vi "WrittingSpectrumAndImageAttributes.vi"() -> ()   [LabVIEW 2009]
uses:
  tango_lv8/tango_vi.llb/WriteBooleanSpectrumAttribute.vi
  tango_lv8/tango_vi.llb/WriteUShortSpectrumAttribute.vi
  tango_lv8/tango_vi.llb/WriteShortSpectrumAttribute.vi
  tango_lv8/tango_vi.llb/WriteUCharSpectrumAttribute.vi
  tango_lv8/tango_vi.llb/ReadShortImageAttribute.vi
  tango_lv8/tango_vi.llb/WriteShortImageAttribute.vi
  tango_lv8/tango_vi.llb/WriteFloatSpectrumAttribute.vi
  tango_lv8/tango_vi.llb/WriteDoubleSpectrumAttribute.vi
  tango_lv8/tango_vi.llb/WriteLongSpectrumAttribute.vi
  tango_lv8/tango_vi.llb/ReadLongImageAttribute.vi
  tango_lv8/tango_vi.llb/WriteLongImageAttribute.vi
  tango_lv8/tango_vi.llb/ReadUShortImageAttribute.vi
  tango_lv8/tango_vi.llb/WriteUShortImageAttribute.vi
  tango_lv8/tango_vi.llb/ReadUCharImageAttribute.vi
  tango_lv8/tango_vi.llb/WriteUCharImageAttribute.vi
  tango_lv8/tango_vi.llb/ReadBooleanImageAttribute.vi
  tango_lv8/tango_vi.llb/WriteBooleanImageAttribute.vi
  tango_lv8/tango_vi.llb/ReadFloatImageAttribute.vi
  tango_lv8/tango_vi.llb/WriteFloatImageAttribute.vi
  tango_lv8/tango_vi.llb/ReadDoubleImageAttribute.vi
  tango_lv8/tango_vi.llb/WriteDoubleImageAttribute.vi
  tango_lv8/tango_vi.llb/ReadBooleanSpectrumAttribute.vi
  tango_lv8/tango_vi.llb/ReadUCharSpectrumAttribute.vi
  tango_lv8/tango_vi.llb/ReadUShortSpectrumAttribute.vi
  tango_lv8/tango_vi.llb/ReadShortSpectrumAttribute.vi
  tango_lv8/tango_vi.llb/ReadFloatSpectrumAttribute.vi
  tango_lv8/tango_vi.llb/ReadDoubleSpectrumAttribute.vi
  tango_lv8/tango_vi.llb/ReadLongSpectrumAttribute.vi
  tango_lv8/tango_vi.llb/ReadULongImageAttribute.vi
  tango_lv8/tango_vi.llb/WriteULongImageAttribute.vi
  tango_lv8/tango_vi.llb/WriteULongSpectrumAttribute.vi
  tango_lv8/tango_vi.llb/ReadULongSpectrumAttribute.vi
panel:
  out "ULong Spectrum R":u32[](graph)
  out "Success-R":bool
  out "Success-Cmp 4":bool
  out "Success-W":bool
  out "ULong  Spectrum W":u32[](graph)
  in  "TangoTest dev. name 3":string="tango/tangotest/1"
  out "Success-R":bool
  out "Success-Cmp 3":bool
  out "ULong Image R":u32[][](graph)
  out "Success-W":bool
  out "ULong Image W":u32[][](graph)
  out "Success-R":bool
  out "Success-Cmp":bool
  out "Double  Image R":dbl[][](graph)
  out "Success-W":bool
  out "Double Image W":dbl[][](graph)
  out "Success-R":bool
  out "Success-Cmp":bool
  out "Float Image R":sgl[][](graph)
  out "Success-W":bool
  out "Float Image W":sgl[][](graph)
  out "Success-R":bool
  out "Success-Cmp":bool
  out "Boolean  Image R":i16[][](graph)
  out "Success-W":bool
  out "Boolean Image W":i16[][](graph)
  out "Success-R":bool
  out "Success-Cmp":bool
  out "UChar Image R":u8[][](graph)
  out "Success-W":bool
  out "UChar Image W":u8[][](graph)
  out "Success-R":bool
  out "Success-Cmp":bool
  out "UShort Image R":u16[][](graph)
  out "Success-W":bool
  out "UShort Image W":u16[][](graph)
  out "Long Spectrum R":i32[](graph)
  out "Success-R":bool
  out "Success-Cmp":bool
  out "Success-W":bool
  out "Long  Spectrum W":i32[](graph)
  out "Success-R":bool
  out "Success-Cmp":bool
  out "Long Image R":i32[][](graph)
  out "Success-W":bool
  out "Long Image W":i32[][](graph)
  out "Double Spectrum R":dbl[](graph)
  out "Success-R":bool
  out "Success-Cmp":bool
  out "Success-W":bool
  out "Double  Spectrum W":dbl[](graph)
  out "Float Spectrum R":sgl[](graph)
  out "Success-R":bool
  out "Success-Cmp":bool
  out "Success-W":bool
  out "Float Spectrum W":sgl[](graph)
  out "Short Image R":i16[][](graph)
  out "Short Image W":i16[][](graph)
  out "Success-R":bool
  out "Success-Cmp 2":bool
  out "Success-W":bool
  out "error stack":string[](array[string])
  in  "TangoTest Device Name 5":string="tango/tangotest/1"
  in  "TangoTest Device Name 4":string="tango/tangotest/1"
  in  "TangoTest Device Name 3":string="tango/tangotest/1"
  in  "TangoTest Device Name 2":string="tango/tangotest/1"
  in  "TangoTest dev. name":string="tango/tangotest/1"
  out "UChar Spectrum R":u8[](graph)
  out "Success-R":bool
  out "Success-Cmp":bool
  out "Success-W":bool
  out "UChar Spectrum W":u8[](graph)
  out "Boolean Spectrum R":i16[](graph)
  out "Success-R":bool
  out "Success-Cmp":bool
  out "Success-W":bool
  out "Boolean Spectrum W":i16[](graph)
  out "UShort Spectrum R":u16[](graph)
  out "Success-R":bool
  out "Success-Cmp":bool
  out "Success-W":bool
  out "UShort Spectrum W":u16[](graph)
  out "Success-Cmp":bool
  out "Success-W":bool
  out "Short Spectrum R":i16[](graph)
  out "Success-R":bool
  out "Short Spectrum W":i16[](graph)
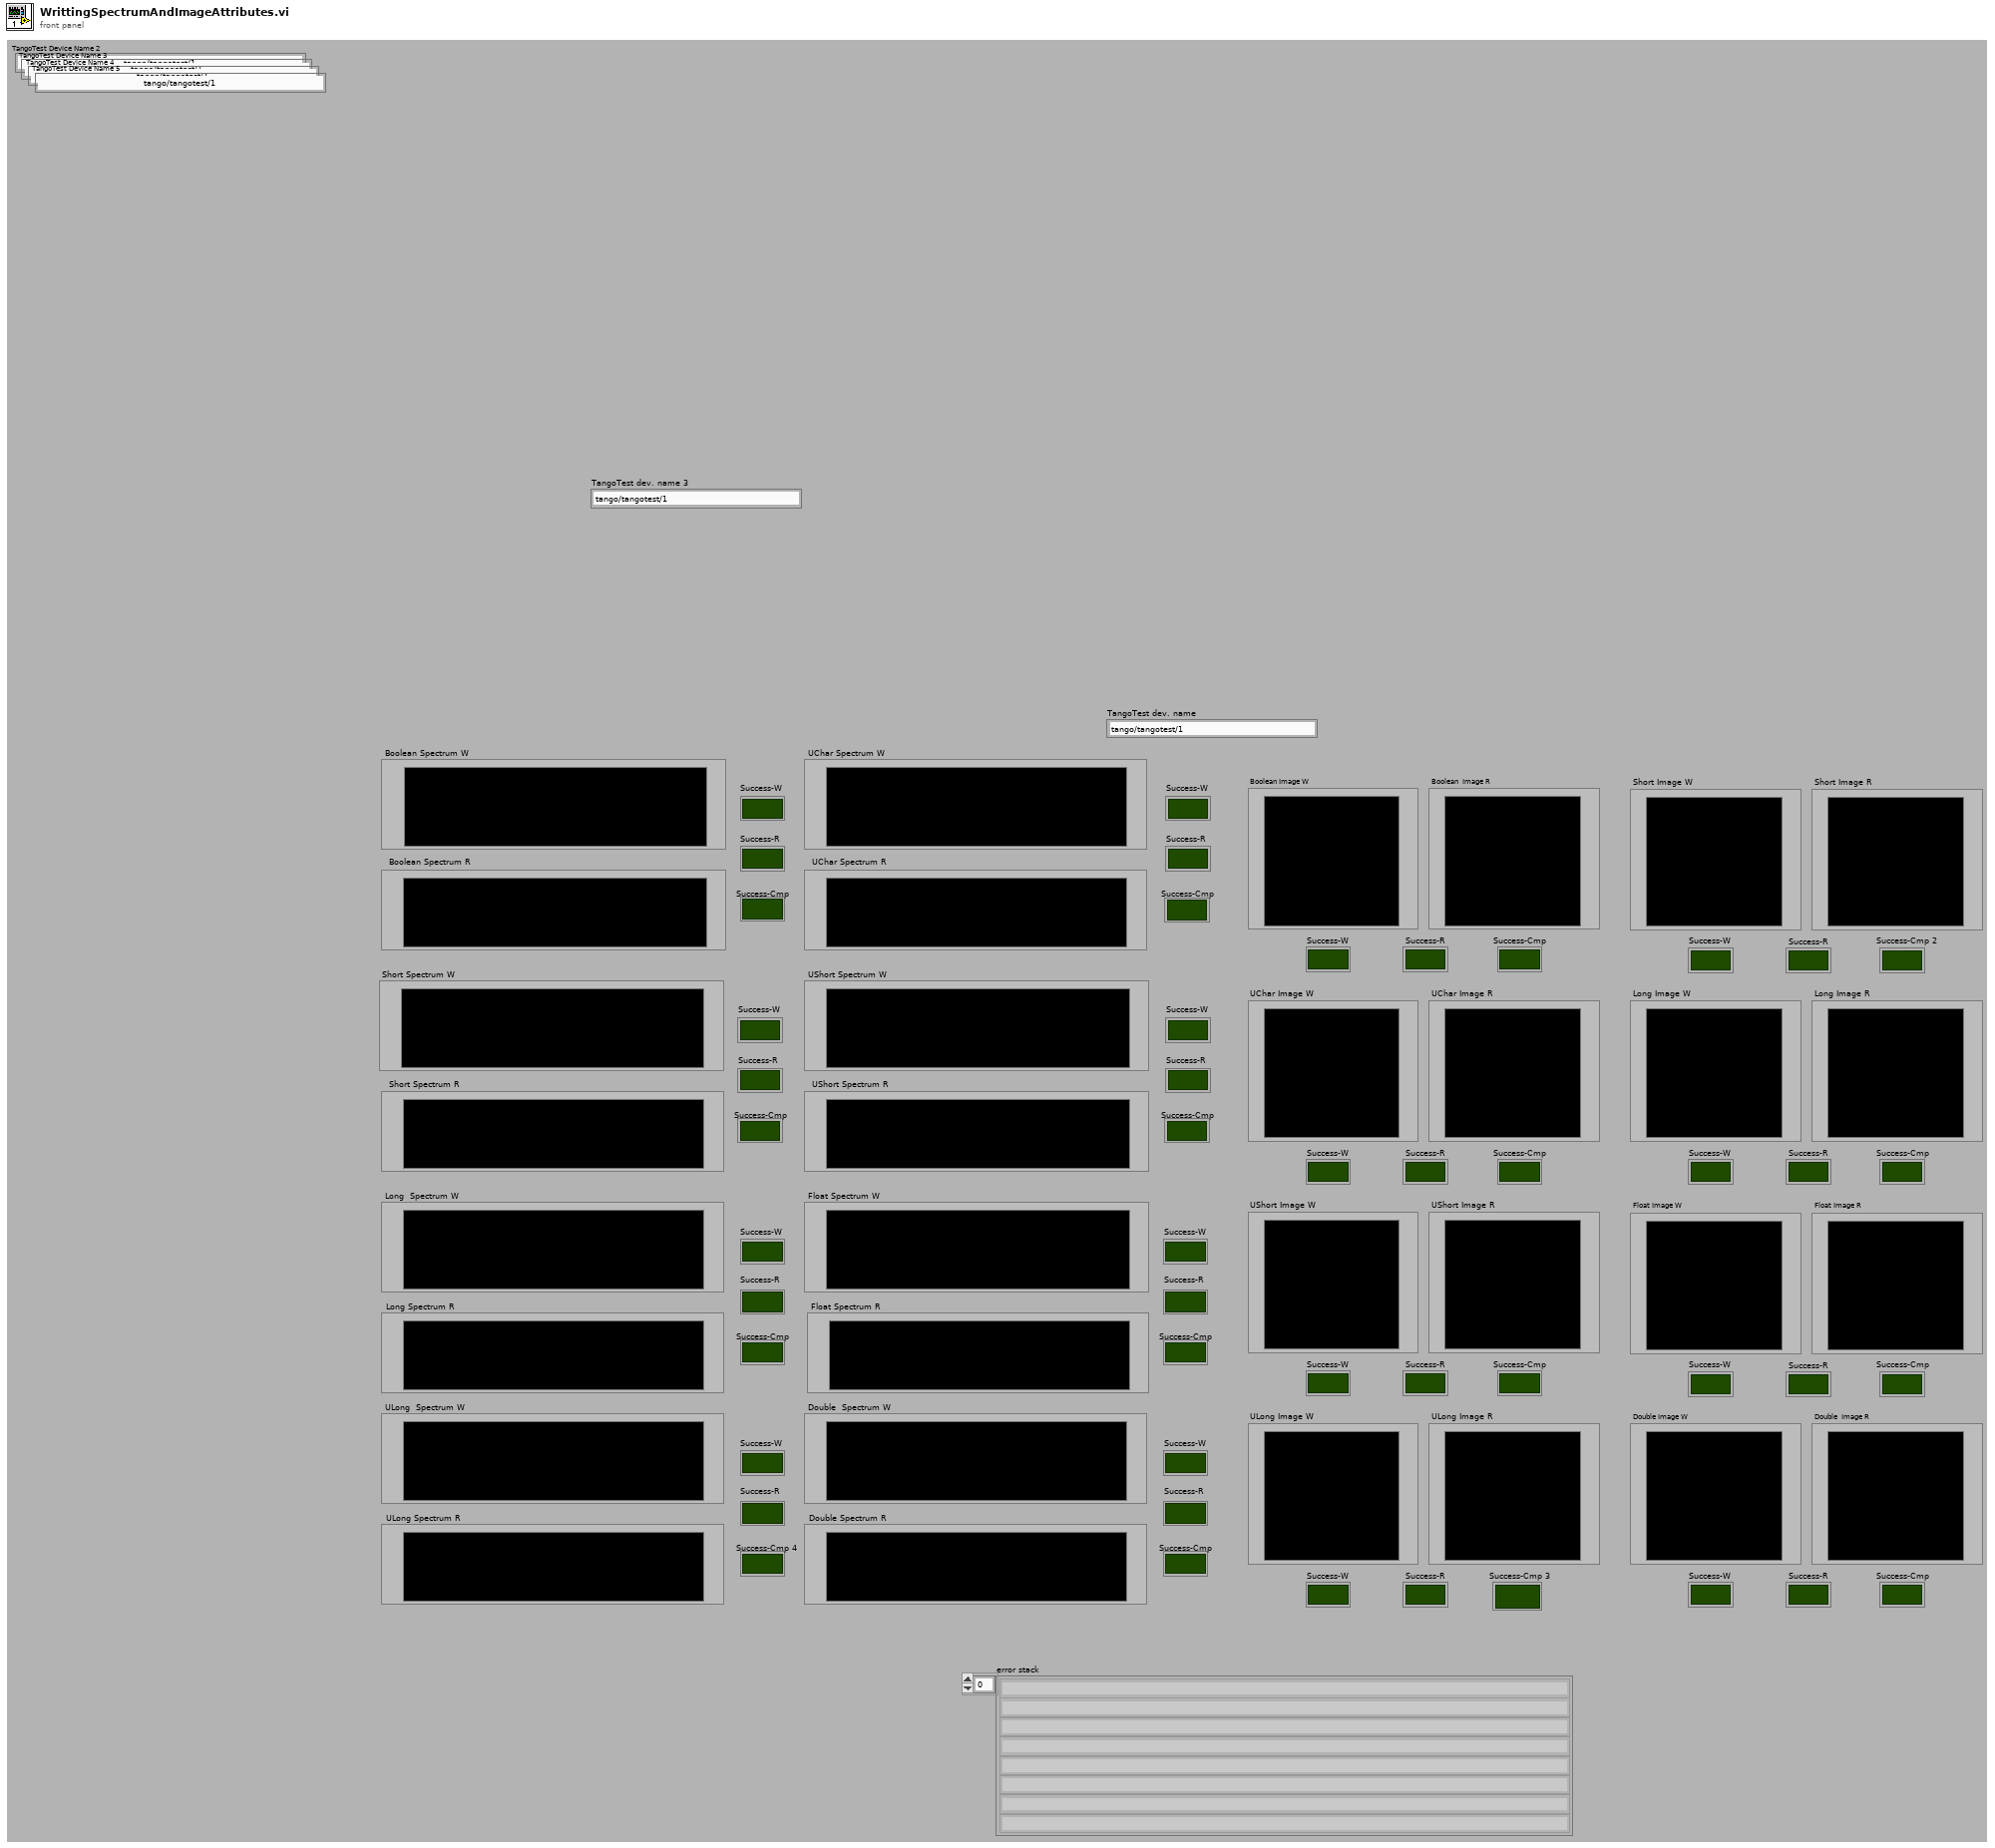
[diagram p1: front panel]
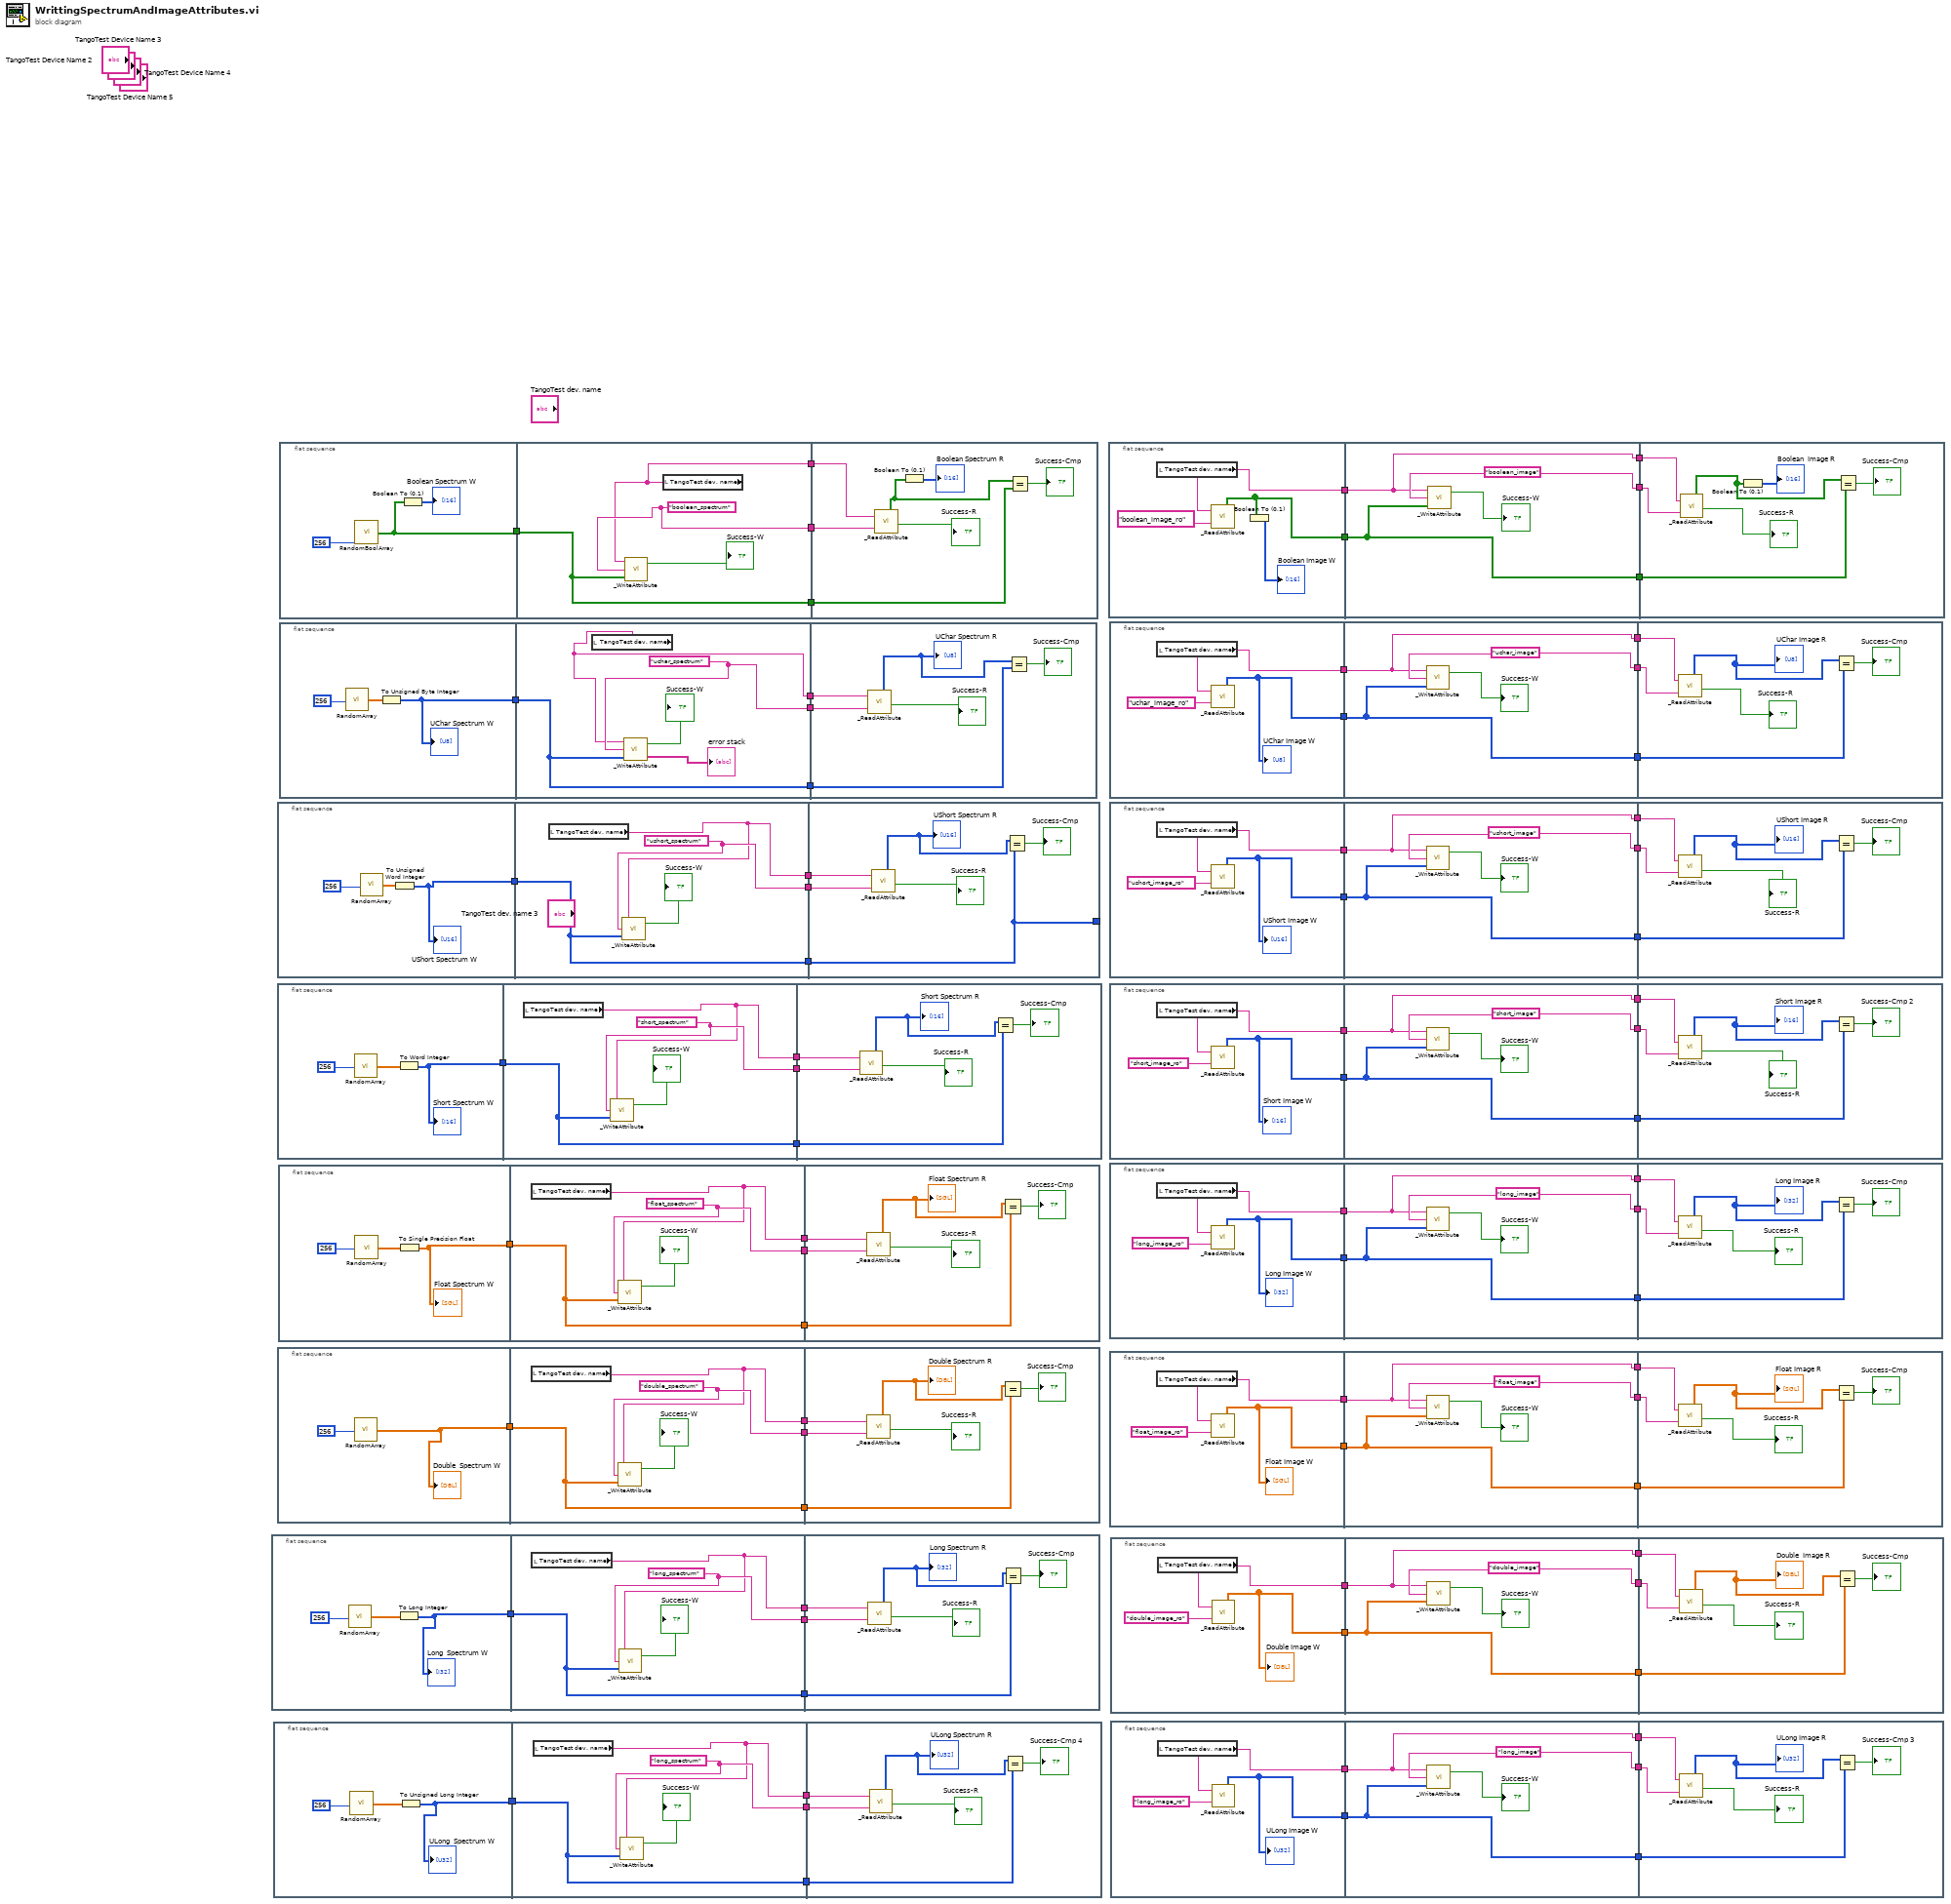
[diagram p0: block diagram]
diagram:
  n1 = flat-sequence {
    tunnel: [w73] -> w38
    tunnel: [w76] -> w37
    tunnel: [w78] -> w36
    tunnel: [w77] -> w35
    tunnel: w38 -> [w77]
    tunnel: w37 -> [w84]
    tunnel: w36 -> [w83]
    tunnel: w35 -> [w81]
    frame #0 {
      n2 = call "RandomArray.vi"("random array size"=256) -> ("random array"=w74:dbl[])  [unwired: 1 in]
      n3 = To Long Integer(number=w74) -> (32bit integer=w73:i32[])
      "Long  Spectrum W" <- w73
    }
    frame #1 {
      w78 = "long_spectrum" ("attribute name")
      n4 = local read "TangoTest dev. name"() -> (w76:string)
      n5 = call-poly "_WriteAttribute.vi"("value"=w77, "attribute name"=w78, "device name"=w76) -> ("success"=→"Success-W":bool)  [unwired: 1 out]
    }
    frame #2 {
      n6 = call-poly "_ReadAttribute.vi"("device name"=w84, "attribute name"=w83) -> ("value"=w82:i32[], "success"=→"Success-R":bool)  [unwired: 4 out]
      "Long Spectrum R" <- w82
      n7 = Equal?(x=w82, y=w81) -> (x = y?=→"Success-Cmp":bool)
    }
  }
  n8 = flat-sequence {
    tunnel: [w86] -> w4
    tunnel: [w89] -> w3
    tunnel: [w91] -> w2
    tunnel: [w90] -> w1
    tunnel: w4 -> [w90]
    tunnel: w3 -> [w97]
    tunnel: w2 -> [w96]
    tunnel: w1 -> [w94]
    frame #0 {
      n9 = call "RandomArray.vi"("random array size"=256) -> ("random array"=w87:dbl[])  [unwired: 1 in]
      n10 = To Unsigned Long Integer(number=w87) -> (unsigned 32bit integer=w86:u32[])
      "ULong  Spectrum W" <- w86
    }
    frame #1 {
      w91 = "long_spectrum" ("attribute name")
      n11 = local read "TangoTest dev. name"() -> (w89:string)
      n12 = call-poly "_WriteAttribute.vi"("value"=w90, "attribute name"=w91, "device name"=w89) -> ("success"=→"Success-W":bool)  [unwired: 1 out]
    }
    frame #2 {
      n13 = call-poly "_ReadAttribute.vi"("device name"=w97, "attribute name"=w96) -> ("value"=w95:u32[], "success"=→"Success-R":bool)  [unwired: 4 out]
      "ULong Spectrum R" <- w95
      n14 = Equal?(x=w95, y=w94) -> (x = y?=→"Success-Cmp 4":bool)
    }
  }
  n15 = flat-sequence {
    tunnel: [w99] -> w68
    tunnel: [w102] -> w67
    tunnel: [w104] -> w66
    tunnel: [w103] -> w65
    tunnel: w68 -> [w103]
    tunnel: w67 -> [w110]
    tunnel: w66 -> [w109]
    tunnel: w65 -> [w106]
    tunnel: [w106] -> _
    frame #0 {
      n16 = call "RandomArray.vi"("random array size"=256) -> ("random array"=w100:dbl[])  [unwired: 1 in]
      n17 = To Unsigned Word Integer(number=w100) -> (unsigned 16bit integer=w99:u16[])
      "UShort Spectrum W" <- w99
    }
    frame #1 {
      w104 = "ushort_spectrum" ("attribute name")
      n18 = local read "TangoTest dev. name"() -> (w102:string)
      n19 = call-poly "_WriteAttribute.vi"("value"=w103, "attribute name"=w104, "device name"=w102) -> ("success"=→"Success-W":bool)  [unwired: 1 out]
    }
    frame #2 {
      n20 = call-poly "_ReadAttribute.vi"("device name"=w110, "attribute name"=w109) -> ("value"=w108:u16[], "success"=→"Success-R":bool)  [unwired: 4 out]
      "UShort Spectrum R" <- w108
      n21 = Equal?(x=w108, y=w106) -> (x = y?=→"Success-Cmp":bool)
    }
  }
  n22 = flat-sequence {
    tunnel: [w112] -> w69
    tunnel: [w115] -> w72
    tunnel: [w117] -> w71
    tunnel: [w116] -> w70
    tunnel: w69 -> [w116]
    tunnel: w72 -> [w123]
    tunnel: w71 -> [w122]
    tunnel: w70 -> [w120]
    frame #0 {
      n23 = call "RandomArray.vi"("random array size"=256) -> ("random array"=w113:dbl[])  [unwired: 1 in]
      n24 = To Word Integer(number=w113) -> (16bit integer=w112:i16[])
      "Short Spectrum W" <- w112
    }
    frame #1 {
      w117 = "short_spectrum" ("attribute name")
      n25 = local read "TangoTest dev. name"() -> (w115:string)
      n26 = call-poly "_WriteAttribute.vi"("value"=w116, "attribute name"=w117, "device name"=w115) -> ("success"=→"Success-W":bool)  [unwired: 1 out]
    }
    frame #2 {
      n27 = call-poly "_ReadAttribute.vi"("device name"=w123, "attribute name"=w122) -> ("value"=w121:i16[], "success"=→"Success-R":bool)  [unwired: 4 out]
      "Short Spectrum R" <- w121
      n28 = Equal?(x=w121, y=w120) -> (x = y?=→"Success-Cmp":bool)
    }
  }
  n29 = flat-sequence {
    tunnel: [w125] -> w47
    tunnel: [w127] -> w46
    tunnel: [w129] -> w45
    tunnel: [w128] -> w44
    tunnel: w47 -> [w128]
    tunnel: w46 -> [w135]
    tunnel: w45 -> [w134]
    tunnel: w44 -> [w132]
    frame #0 {
      n30 = call "RandomArray.vi"("random array size"=256) -> ("random array"=w125:dbl[])  [unwired: 1 in]
      "Double  Spectrum W" <- w125
    }
    frame #1 {
      w129 = "double_spectrum" ("attribute name")
      n31 = local read "TangoTest dev. name"() -> (w127:string)
      n32 = call-poly "_WriteAttribute.vi"("value"=w128, "attribute name"=w129, "device name"=w127) -> ("success"=→"Success-W":bool)  [unwired: 1 out]
    }
    frame #2 {
      n33 = call-poly "_ReadAttribute.vi"("device name"=w135, "attribute name"=w134) -> ("value"=w133:dbl[], "success"=→"Success-R":bool)  [unwired: 4 out]
      "Double Spectrum R" <- w133
      n34 = Equal?(x=w133, y=w132) -> (x = y?=→"Success-Cmp":bool)
    }
  }
  n35 = flat-sequence {
    tunnel: [w137] -> w51
    tunnel: [w140] -> w50
    tunnel: [w142] -> w49
    tunnel: [w141] -> w48
    tunnel: w51 -> [w141]
    tunnel: w50 -> [w148]
    tunnel: w49 -> [w147]
    tunnel: w48 -> [w145]
    frame #0 {
      n36 = call "RandomArray.vi"("random array size"=256) -> ("random array"=w138:dbl[])  [unwired: 1 in]
      n37 = To Single Precision Float(number=w138) -> (single precision float=w137:sgl[])
      "Float Spectrum W" <- w137
    }
    frame #1 {
      w142 = "float_spectrum" ("attribute name")
      n38 = local read "TangoTest dev. name"() -> (w140:string)
      n39 = call-poly "_WriteAttribute.vi"("value"=w141, "attribute name"=w142, "device name"=w140) -> ("success"=→"Success-W":bool)  [unwired: 1 out]
    }
    frame #2 {
      n40 = call-poly "_ReadAttribute.vi"("device name"=w148, "attribute name"=w147) -> ("value"=w146:sgl[], "success"=→"Success-R":bool)  [unwired: 4 out]
      "Float Spectrum R" <- w146
      n41 = Equal?(x=w146, y=w145) -> (x = y?=→"Success-Cmp":bool)
    }
  }
  n42 = flat-sequence {
    tunnel: [w150] -> w58
    tunnel: [w154] -> w62
    tunnel: [w156] -> w61
    tunnel: w58 -> [w155]
    tunnel: [w155] -> w57
    tunnel: w62 -> [w162]
    tunnel: w61 -> [w161]
    tunnel: w57 -> [w158]
    frame #0 {
      n43 = call "RandomArray.vi"("random array size"=256) -> ("random array"=w151:dbl[])  [unwired: 1 in]
      n44 = To Unsigned Byte Integer(number=w151) -> (unsigned 8bit integer=w150:u8[])
      "UChar Spectrum W" <- w150
    }
    frame #1 {
      w156 = "uchar_spectrum" ("attribute name")
      n45 = local read "TangoTest dev. name"() -> (w154:string)
      n46 = call-poly "_WriteAttribute.vi"("value"=w155, "attribute name"=w156, "device name"=w154) -> ("error stack"=→"error stack":string[], "success"=→"Success-W":bool)
    }
    frame #2 {
      n47 = call-poly "_ReadAttribute.vi"("device name"=w162, "attribute name"=w161) -> ("value"=w160:u8[], "success"=→"Success-R":bool)  [unwired: 4 out]
      "UChar Spectrum R" <- w160
      n48 = Equal?(x=w160, y=w158) -> (x = y?=→"Success-Cmp":bool)
    }
  }
  n49 = flat-sequence {
    tunnel: [w165] -> w64
    tunnel: [w169] -> w63
    tunnel: w64 -> [w169]
    tunnel: [w168] -> w60
    tunnel: [w167] -> w59
    tunnel: w63 -> [w173]
    tunnel: w60 -> [w172]
    tunnel: w59 -> [w171]
    frame #0 {
      n50 = call "RandomBoolArray.vi"("random array size"=256) -> ("random array"=w165:bool[])  [unwired: 1 in]
      n51 = Boolean To (0,1)(Boolean=w165) -> (0, 1=→"Boolean Spectrum W":i16[])
    }
    frame #1 {
      w168 = "boolean_spectrum" ("attribute name")
      n52 = local read "TangoTest dev. name"() -> (w167:string)
      n53 = call-poly "_WriteAttribute.vi"("value"=w169, "attribute name"=w168, "device name"=w167) -> ("success"=→"Success-W":bool)  [unwired: 1 out]
    }
    frame #2 {
      n54 = call-poly "_ReadAttribute.vi"("device name"=w171, "attribute name"=w172) -> ("value"=w175:bool[], "success"=→"Success-R":bool)  [unwired: 4 out]
      n55 = Boolean To (0,1)(Boolean=w175) -> (0, 1=→"Boolean Spectrum R":i16[])
      n56 = Equal?(x=w175, y=w173) -> (x = y?=→"Success-Cmp":bool)
    }
  }
  n57 = flat-sequence {
    tunnel: [w180] -> w24
    tunnel: [w179] -> w23
    tunnel: [w185] -> w22
    tunnel: [w183] -> w21
    tunnel: w24 -> [w183]
    tunnel: w23 -> [w182]
    tunnel: [w182] -> w20
    tunnel: w22 -> [w191]
    tunnel: w21 -> [w188]
    tunnel: w20 -> [w187]
    frame #0 {
      n58 = local read "TangoTest dev. name"() -> (w179:string)
      n59 = call-poly "_ReadAttribute.vi"("device name"=w179, "attribute name"="boolean_image_ro") -> ("value"=w180:bool[][])  [unwired: 5 out]
      n60 = Boolean To (0,1)(Boolean=w180) -> (0, 1=→"Boolean Image W":i16[][])
    }
    frame #1 {
      w185 = "boolean_image" ("attribute name")
      n61 = call-poly "_WriteAttribute.vi"("value"=w183, "attribute name"=w185, "device name"=w182) -> ("success"=→"Success-W":bool)  [unwired: 1 out]
    }
    frame #2 {
      n62 = call-poly "_ReadAttribute.vi"("device name"=w187, "attribute name"=w191) -> ("value"=w189:bool[][], "success"=→"Success-R":bool)  [unwired: 4 out]
      n63 = Boolean To (0,1)(Boolean=w189) -> (0, 1=→"Boolean  Image R":i16[][])
      n64 = Equal?(x=w189, y=w188) -> (x = y?=→"Success-Cmp":bool)
    }
  }
  n65 = flat-sequence {
    tunnel: [w194] -> w29
    tunnel: [w193] -> w28
    tunnel: [w199] -> w27
    tunnel: [w197] -> w26
    tunnel: w29 -> [w197]
    tunnel: w28 -> [w196]
    tunnel: [w196] -> w25
    tunnel: w27 -> [w204]
    tunnel: w26 -> [w201]
    tunnel: w25 -> [w200]
    frame #0 {
      n66 = local read "TangoTest dev. name"() -> (w193:string)
      n67 = call-poly "_ReadAttribute.vi"("device name"=w193, "attribute name"="uchar_image_ro") -> ("value"=w194:u8[][])  [unwired: 5 out]
      "UChar Image W" <- w194
    }
    frame #1 {
      w199 = "uchar_image" ("attribute name")
      n68 = call-poly "_WriteAttribute.vi"("value"=w197, "attribute name"=w199, "device name"=w196) -> ("success"=→"Success-W":bool)  [unwired: 1 out]
    }
    frame #2 {
      n69 = call-poly "_ReadAttribute.vi"("device name"=w200, "attribute name"=w204) -> ("value"=w202:u8[][], "success"=→"Success-R":bool)  [unwired: 4 out]
      "UChar Image R" <- w202
      n70 = Equal?(x=w202, y=w201) -> (x = y?=→"Success-Cmp":bool)
    }
  }
  n71 = flat-sequence {
    tunnel: [w207] -> w34
    tunnel: [w206] -> w33
    tunnel: [w212] -> w32
    tunnel: [w210] -> w31
    tunnel: w34 -> [w210]
    tunnel: w33 -> [w209]
    tunnel: [w209] -> w30
    tunnel: w32 -> [w217]
    tunnel: w31 -> [w214]
    tunnel: w30 -> [w213]
    frame #0 {
      n72 = local read "TangoTest dev. name"() -> (w206:string)
      n73 = call-poly "_ReadAttribute.vi"("device name"=w206, "attribute name"="ushort_image_ro") -> ("value"=w207:u16[][])  [unwired: 5 out]
      "UShort Image W" <- w207
    }
    frame #1 {
      w212 = "ushort_image" ("attribute name")
      n74 = call-poly "_WriteAttribute.vi"("value"=w210, "attribute name"=w212, "device name"=w209) -> ("success"=→"Success-W":bool)  [unwired: 1 out]
    }
    frame #2 {
      n75 = call-poly "_ReadAttribute.vi"("device name"=w213, "attribute name"=w217) -> ("value"=w215:u16[][], "success"=→"Success-R":bool)  [unwired: 4 out]
      "UShort Image R" <- w215
      n76 = Equal?(x=w215, y=w214) -> (x = y?=→"Success-Cmp":bool)
    }
  }
  n77 = flat-sequence {
    tunnel: [w220] -> w54
    tunnel: [w219] -> w53
    tunnel: [w225] -> w56
    tunnel: [w223] -> w55
    tunnel: w54 -> [w223]
    tunnel: w53 -> [w222]
    tunnel: [w222] -> w52
    tunnel: w56 -> [w230]
    tunnel: w55 -> [w227]
    tunnel: w52 -> [w226]
    frame #0 {
      n78 = local read "TangoTest dev. name"() -> (w219:string)
      n79 = call-poly "_ReadAttribute.vi"("device name"=w219, "attribute name"="short_image_ro") -> ("value"=w220:i16[][])  [unwired: 5 out]
      "Short Image W" <- w220
    }
    frame #1 {
      w225 = "short_image" ("attribute name")
      n80 = call-poly "_WriteAttribute.vi"("value"=w223, "attribute name"=w225, "device name"=w222) -> ("success"=→"Success-W":bool)  [unwired: 1 out]
    }
    frame #2 {
      n81 = call-poly "_ReadAttribute.vi"("device name"=w226, "attribute name"=w230) -> ("value"=w228:i16[][], "success"=→"Success-R":bool)  [unwired: 4 out]
      "Short Image R" <- w228
      n82 = Equal?(x=w228, y=w227) -> (x = y?=→"Success-Cmp 2":bool)
    }
  }
  n83 = flat-sequence {
    tunnel: [w233] -> w43
    tunnel: [w232] -> w42
    tunnel: [w238] -> w41
    tunnel: [w236] -> w40
    tunnel: w43 -> [w236]
    tunnel: w42 -> [w235]
    tunnel: [w235] -> w39
    tunnel: w41 -> [w243]
    tunnel: w40 -> [w240]
    tunnel: w39 -> [w239]
    frame #0 {
      n84 = local read "TangoTest dev. name"() -> (w232:string)
      n85 = call-poly "_ReadAttribute.vi"("device name"=w232, "attribute name"="long_image_ro") -> ("value"=w233:i32[][])  [unwired: 5 out]
      "Long Image W" <- w233
    }
    frame #1 {
      w238 = "long_image" ("attribute name")
      n86 = call-poly "_WriteAttribute.vi"("value"=w236, "attribute name"=w238, "device name"=w235) -> ("success"=→"Success-W":bool)  [unwired: 1 out]
    }
    frame #2 {
      n87 = call-poly "_ReadAttribute.vi"("device name"=w239, "attribute name"=w243) -> ("value"=w241:i32[][], "success"=→"Success-R":bool)  [unwired: 4 out]
      "Long Image R" <- w241
      n88 = Equal?(x=w241, y=w240) -> (x = y?=→"Success-Cmp":bool)
    }
  }
  n89 = flat-sequence {
    tunnel: [w246] -> w19
    tunnel: [w245] -> w18
    tunnel: [w251] -> w17
    tunnel: [w249] -> w16
    tunnel: w19 -> [w249]
    tunnel: w18 -> [w248]
    tunnel: [w248] -> w15
    tunnel: w17 -> [w256]
    tunnel: w16 -> [w253]
    tunnel: w15 -> [w252]
    frame #0 {
      n90 = local read "TangoTest dev. name"() -> (w245:string)
      n91 = call-poly "_ReadAttribute.vi"("device name"=w245, "attribute name"="float_image_ro") -> ("value"=w246:sgl[][])  [unwired: 5 out]
      "Float Image W" <- w246
    }
    frame #1 {
      w251 = "float_image" ("attribute name")
      n92 = call-poly "_WriteAttribute.vi"("value"=w249, "attribute name"=w251, "device name"=w248) -> ("success"=→"Success-W":bool)  [unwired: 1 out]
    }
    frame #2 {
      n93 = call-poly "_ReadAttribute.vi"("device name"=w252, "attribute name"=w256) -> ("value"=w254:sgl[][], "success"=→"Success-R":bool)  [unwired: 4 out]
      "Float Image R" <- w254
      n94 = Equal?(x=w254, y=w253) -> (x = y?=→"Success-Cmp":bool)
    }
  }
  n95 = flat-sequence {
    tunnel: [w259] -> w14
    tunnel: [w258] -> w13
    tunnel: [w264] -> w12
    tunnel: [w262] -> w11
    tunnel: w14 -> [w262]
    tunnel: w13 -> [w261]
    tunnel: [w261] -> w10
    tunnel: w12 -> [w269]
    tunnel: w11 -> [w266]
    tunnel: w10 -> [w265]
    frame #0 {
      n96 = local read "TangoTest dev. name"() -> (w258:string)
      n97 = call-poly "_ReadAttribute.vi"("device name"=w258, "attribute name"="double_image_ro") -> ("value"=w259:dbl[][])  [unwired: 5 out]
      "Double Image W" <- w259
    }
    frame #1 {
      w264 = "double_image" ("attribute name")
      n98 = call-poly "_WriteAttribute.vi"("value"=w262, "attribute name"=w264, "device name"=w261) -> ("success"=→"Success-W":bool)  [unwired: 1 out]
    }
    frame #2 {
      n99 = call-poly "_ReadAttribute.vi"("device name"=w265, "attribute name"=w269) -> ("value"=w267:dbl[][], "success"=→"Success-R":bool)  [unwired: 4 out]
      "Double  Image R" <- w267
      n100 = Equal?(x=w267, y=w266) -> (x = y?=→"Success-Cmp":bool)
    }
  }
  n101 = flat-sequence {
    tunnel: [w272] -> w9
    tunnel: [w271] -> w8
    tunnel: [w277] -> w7
    tunnel: [w275] -> w6
    tunnel: w9 -> [w275]
    tunnel: w8 -> [w274]
    tunnel: [w274] -> w5
    tunnel: w7 -> [w282]
    tunnel: w6 -> [w279]
    tunnel: w5 -> [w278]
    frame #0 {
      n102 = local read "TangoTest dev. name"() -> (w271:string)
      n103 = call-poly "_ReadAttribute.vi"("device name"=w271, "attribute name"="long_image_ro") -> ("value"=w272:u32[][])  [unwired: 5 out]
      "ULong Image W" <- w272
    }
    frame #1 {
      w277 = "long_image" ("attribute name")
      n104 = call-poly "_WriteAttribute.vi"("value"=w275, "attribute name"=w277, "device name"=w274) -> ("success"=→"Success-W":bool)  [unwired: 1 out]
    }
    frame #2 {
      n105 = call-poly "_ReadAttribute.vi"("device name"=w278, "attribute name"=w282) -> ("value"=w280:u32[][], "success"=→"Success-R":bool)  [unwired: 4 out]
      "ULong Image R" <- w280
      n106 = Equal?(x=w280, y=w279) -> (x = y?=→"Success-Cmp 3":bool)
    }
  }
